vi "KeepProportionsByScales.vi"(10 "Bounds in":T1, 11 "GraphChart in":refnum<vi>) -> (1 "Width's Height":dbl, 2 "Bounds out":T1, 3 "Width":u32, 4 "Height":u32, 5 "Heights' Width":dbl)   [LabVIEW 2022 SP3, in "PentaPanesLibrary.lvlib" / "PentaPanes.lvclass"]
uses:
  PentaPanes.lvclass
  <vilib>/Utility/miscctls.llb/LVBoundsTypeDef.ctl
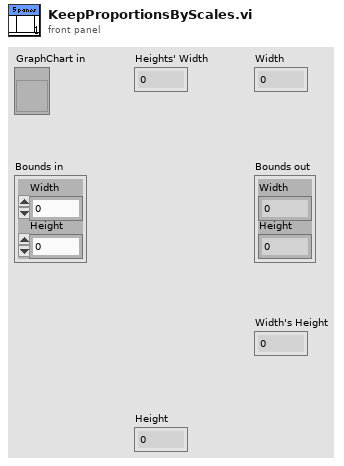
[diagram p1: front panel]
types:
  T1 = typedef "LVBoundsTypeDef.ctl" = cluster{"Width":i32, "Height":i32}
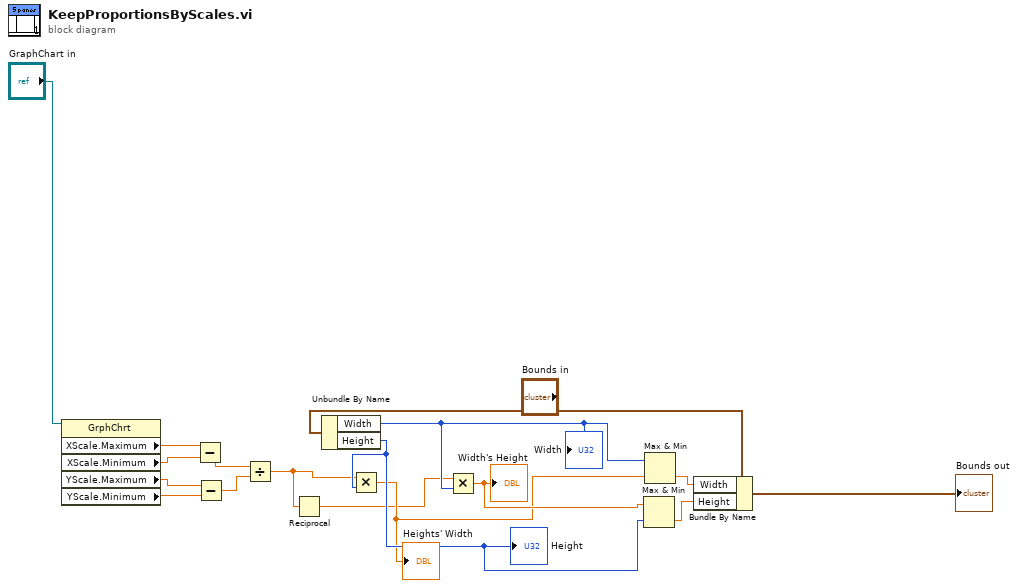
[diagram p0: block diagram]
diagram:
  n1 = property class="GrphChrt"(reference="GraphChart in") -> ("XScale.Maximum"=w2:dbl, "XScale.Minimum"=w3:dbl, "YScale.Maximum"=w4:dbl, "YScale.Minimum"=w5:dbl)  [unwired: 1 in, 2 out]
  n2 = Subtract(x=w2, y=w3) -> (x-y=w6:dbl)
  n3 = Subtract(x=w4, y=w5) -> (x-y=w7:dbl)
  n4 = Divide(x=w6, y=w7) -> (x/y=w8:dbl)
  n5 = Reciprocal(x=w8) -> (1/x=w9:dbl)
  n6 = Unbundle By Name("Bounds in") -> ("Width"=w10:i32, "Height"=w12:i32)
  "Width" <- w10
  "Height" <- w12
  n7 = Multiply(x=w8, y=w12) -> (x*y=w11:dbl)
  "Heights' Width" <- w11
  n8 = Multiply(x=w9, y=w10) -> (x*y=w13:dbl)
  "Width's Height" <- w13
  n9 = Max & Min(x=w13, y=w12) -> (min(x,y)=w15:dbl)  [unwired: 1 out]
  n10 = Max & Min(x=w10, y=w11) -> (min(x,y)=w16:dbl)  [unwired: 1 out]
  n11 = Bundle By Name(cluster="Bounds in", "Width"=w16, "Height"=w15) -> (→"Bounds out":T1)
